vi "Module (Top Level).vi"(8 "error in":errorcluster) -> (0 "error out":errorcluster)   [LabVIEW 2017, in "Controller.lvlib"]
uses:
  Controller.lvlib
  User Events/TypeDefs/Shutdown UE FGV Command.ctl
  Global TypeDefs/Registered Modules.ctl
  Private TypeDefs/Messages.ctl
  Game/Public TypeDefs/Messages.ctl
  mypam/Public TypeDefs/Messages.ctl
  winhost/Public TypeDefs/Messages.ctl
  Private TypeDefs/Event and Data.ctl
  Game/Public TypeDefs/Module Events.ctl
  Game/Libraries/TypeDefs/ClientStatusData.ctl
  mypam/Public TypeDefs/Module Events.ctl
  winhost/Public TypeDefs/Module Events.ctl
  Error Handler/Error Handler.lvlib
  Logger/Logger.lvlib
  Game/Game.lvlib
  mypam/myPAM.lvlib
  WinHost/WinHost.lvlib
  Game/Libraries/GameComms.lvlib
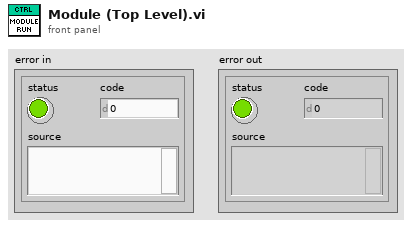
[diagram p1: front panel]
types:
  T1 = typedef "Registered Modules.ctl" = enum16{"Controller", "DAQ", "Error Handler", "Game", "myPAM", "WinHost", "Logger"}
  T2 = typedef "Shutdown UE FGV Command.ctl" = enum16{"create", "get", "destroy"}
  T3 = typedef "WinHost.lvlib/Module Reference.ctl" = cluster{"calling module":T1, "module queues":T4, "module notifiers":T5}
  T4 = typedef "WinHost.lvlib/Module Queues.ctl" = cluster{"message queue":refnum<queue>, "STM queue":refnum<queue>}
  T5 = typedef "WinHost.lvlib/Module Notifiers.ctl" = cluster{"dummy notifier":refnum<notifier>}
  T6 = typedef "myPAM.lvlib/Module Reference.ctl" = cluster{"calling module":T1, "module queues":T7, "module notifiers":T8}
  T7 = typedef "myPAM.lvlib/Module Queues.ctl" = cluster{"message queue":refnum<queue>}
  T8 = typedef "myPAM.lvlib/Module Notifiers.ctl" = cluster{"end eff. pos.":refnum<notifier>}
  T9 = typedef "Game.lvlib/Module Reference.ctl" = cluster{"calling module":T1, "module queues":T10, "module notifiers":T11}
  T10 = typedef "Game.lvlib/Module Queues.ctl" = cluster{"message queue":refnum<queue>}
  T11 = typedef "Game.lvlib/Module Notifiers.ctl" = cluster{"dummy notifier":refnum<notifier>}
  T12 = typedef "Logger.lvlib/Module Reference.ctl" = cluster{"calling module":T1, "module queues":T13, "module notifiers":T14}
  T13 = typedef "Logger.lvlib/Module Queues.ctl" = cluster{"message queue":refnum<queue>}
  T14 = typedef "Logger.lvlib/Module Notifiers.ctl" = cluster{"dummy notifier":refnum<notifier>}
  T15 = typedef "Controller.lvlib/Module Reference.ctl" = cluster{"calling module":T1, "module queues":T16, "module notifiers":T17}
  T16 = typedef "Controller.lvlib/Module Queues.ctl" = cluster{"message queue":refnum<queue>}
  T17 = typedef "Controller.lvlib/Module Notifiers.ctl" = cluster{"dummy notifier":refnum<notifier>}
  T18 = typedef "Error Handler.lvlib/Module Reference.ctl" = cluster{"calling module":T1, "module queues":T19, "module notifiers":T20}
  T19 = typedef "Error Handler.lvlib/Module Queues.ctl" = cluster{"message queue":refnum<queue>}
  T20 = typedef "Error Handler.lvlib/Module Notifiers.ctl" = cluster{"dummy notifier":refnum<notifier>}
  T21 = typedef "Controller.lvlib/Messages.ctl" = enum16{"shutdown", "handle event", "start system"}
  T22 = typedef "myPAM.lvlib/Messages.ctl" = enum16{"calibrate encoders", "enable motors", "disable motors", "operate", "shutdown"}
  T23 = typedef "WinHost.lvlib/Messages.ctl" = enum16{"shutdown", "wait for host", "communicate"}
  T24 = typedef "Game.lvlib/Messages.ctl" = enum16{"wait for client", "communicate", "shutdown"}
  T25 = typedef "Game.lvlib/Module Events.ctl" = enum16{"client connected", "client status change", "client disconnected"}
  T26 = typedef "myPAM.lvlib/Module Events.ctl" = enum16{"critical error"}
  T27 = typedef "WinHost.lvlib/Module Events.ctl" = enum16{"host connected", "enable assistance", "disable assistance", "host disconnected"}
  T28 = typedef "Controller.lvlib/Event and Data.ctl" = cluster{"event":variant, "data":variant}
  T29 = typedef "Game.lvlib/GameComms.lvlib/ClientStatusData.ctl" = cluster{"gameState":u16, "playerName":string, "playerScore":dbl, "gameUnits":string}
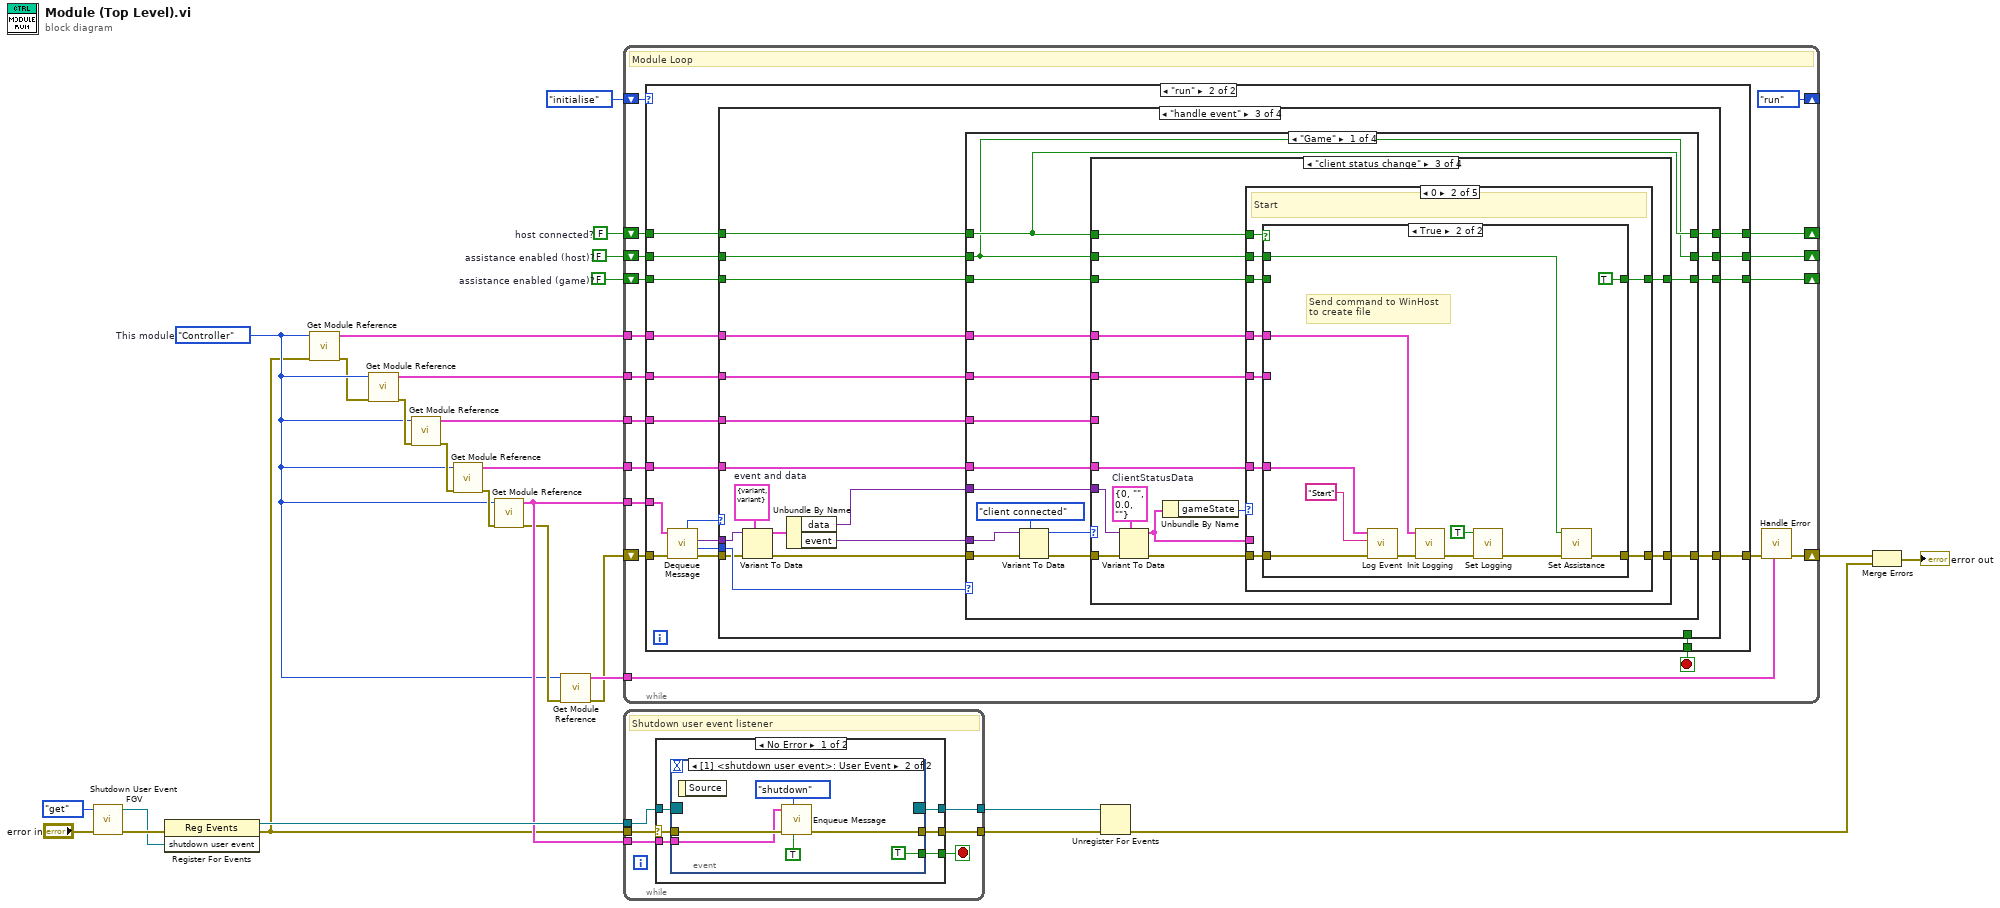
[diagram p0: block diagram]
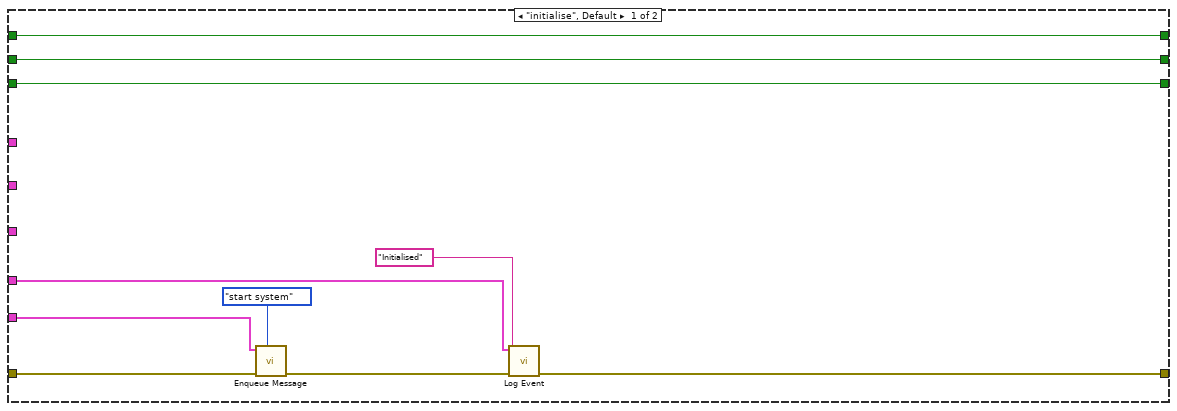
[diagram p2: hidden frame]
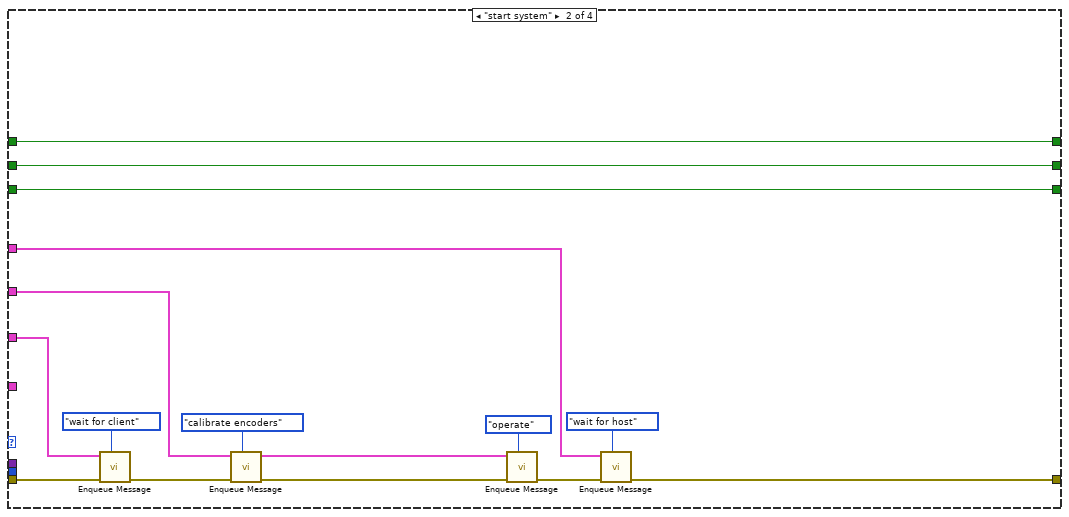
[diagram p4: hidden frame]
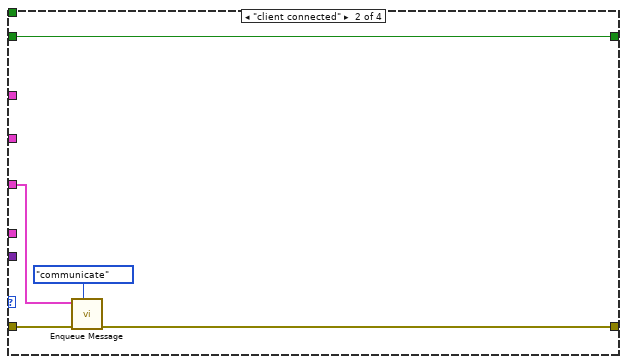
[diagram p6: hidden frame]
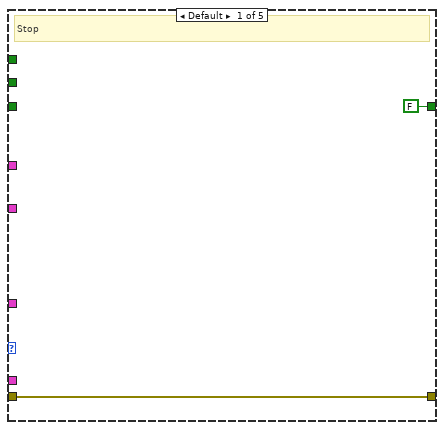
[diagram p7: hidden frame]
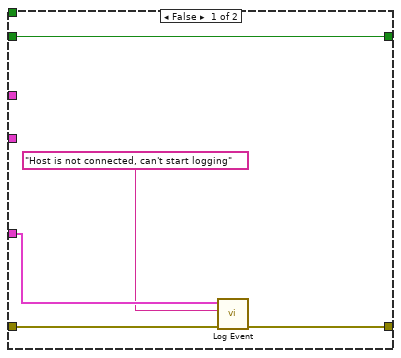
[diagram p8: hidden frame]
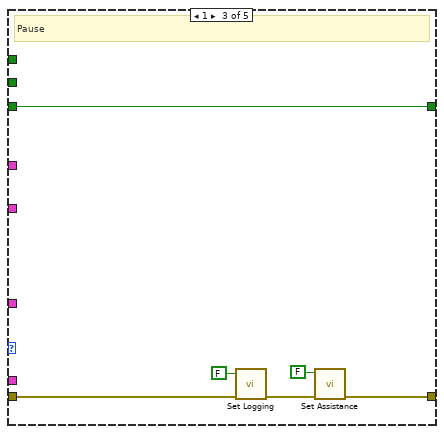
[diagram p9: hidden frame]
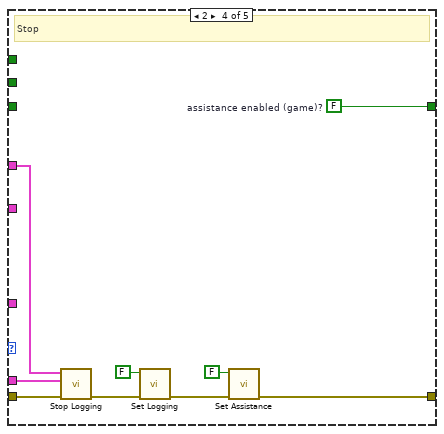
[diagram p10: hidden frame]
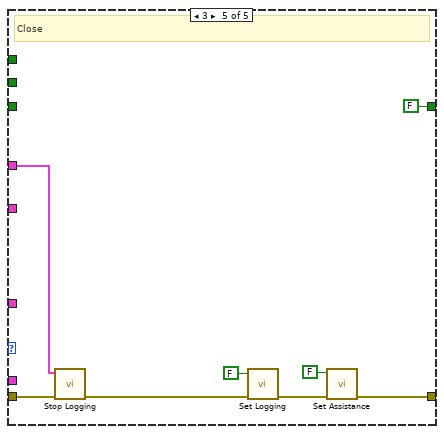
[diagram p11: hidden frame]
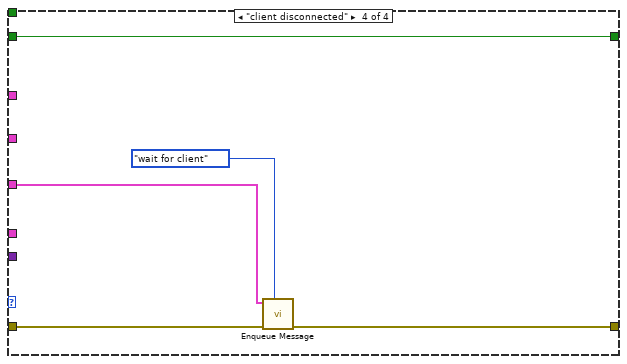
[diagram p12: hidden frame]
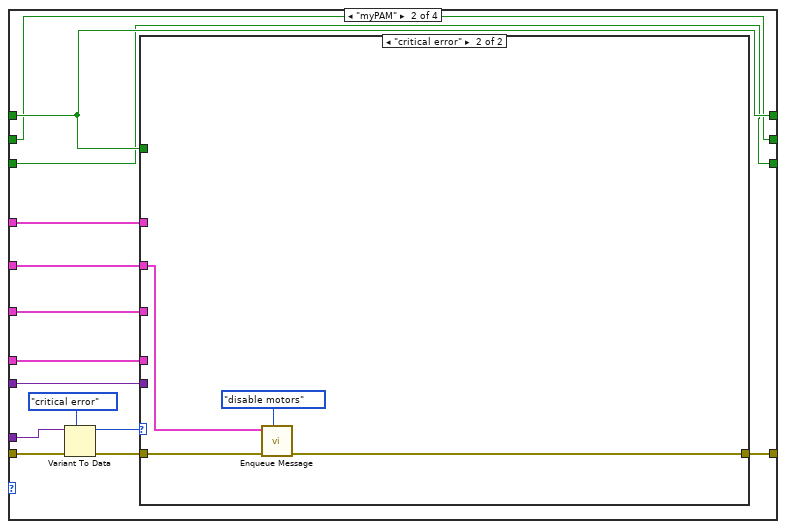
[diagram p13: hidden frame]
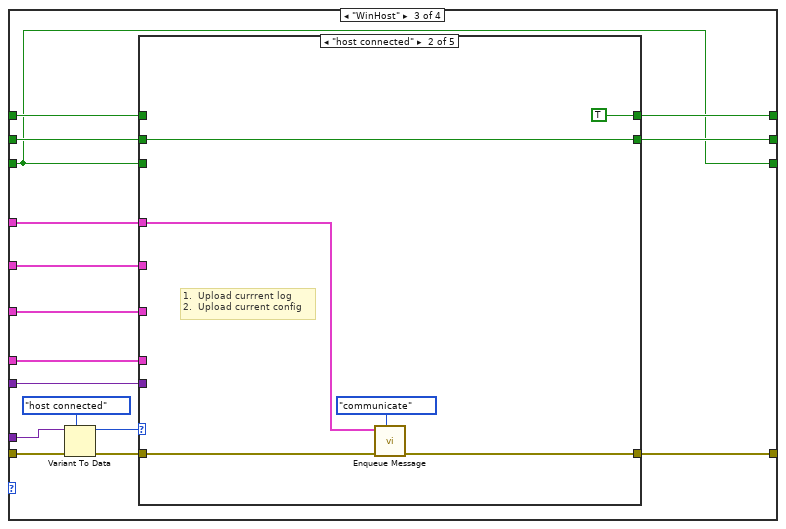
[diagram p15: hidden frame]
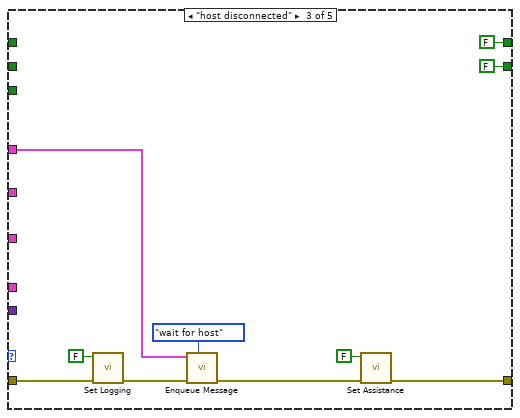
[diagram p17: hidden frame]
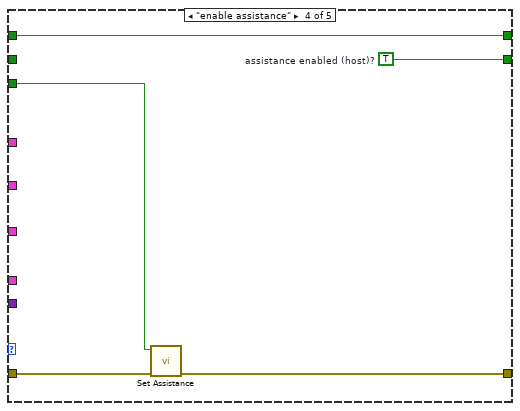
[diagram p18: hidden frame]
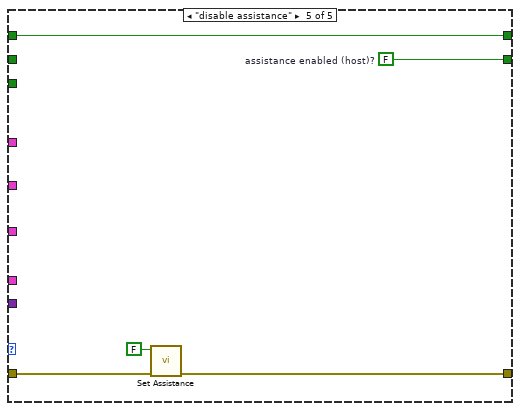
[diagram p19: hidden frame]
diagram:
  w1 = FALSE  # assistance enabled (game)?
  w2 = FALSE  # assistance enabled (host)?
  w4 = FALSE  # host connected?
  w8 = Registered_Modules."Controller"  # This module
  n1 = call "Shutdown User Event FGV.vi"("error in"="error in", "command"=Shutdown_UE_FGV_Command."get" ("Command")) -> ("error out"=w24:errorcluster, "shutdown user event"=w23:refnum<user-event>)  [unwired: 8 in]
  n2 = register-events(error in=w24, w23) -> (reference out=w27:refnum<event-registration>, error out=w7:errorcluster)  [unwired: 1 in]
  n3 = call "Get Module Reference.vi"("error in"=w7, "calling module"=w8) -> ("error out"=w6:errorcluster, "module reference"=w5:T3)  [unwired: 8 in]
  n4 = call "Get Module Reference.vi"("error in"=w6, "calling module"=w8) -> ("error out"=w10:errorcluster, "module reference"=w9:T6)  [unwired: 8 in]
  n5 = call "Get Module Reference.vi"("error in"=w10, "calling module"=w8) -> ("error out"=w12:errorcluster, "module reference"=w11:T9)  [unwired: 8 in]
  n6 = call "Get Module Reference.vi"("error in"=w12, "calling module"=w8) -> ("error out"=w17:errorcluster, "module reference"=w16:T12)  [unwired: 8 in]
  n7 = call "Get Module Reference.vi"("error in"=w17, "calling module"=w8) -> ("error out"=w15:errorcluster, "module reference"=w20:T15)  [unwired: 8 in]
  n8 = call "Get Module Reference.vi"("error in"=w15, "calling module"=w8) -> ("error out"=w13:errorcluster, "module reference"=w14:T18)  [unwired: 8 in]
  n9 = while {
    shift-right: [w40] -> w19
    shift-left: w13 -> [w46]
    tunnel: w20 -> [w45]
    shift-right: [enum16{"initialise", "run"}."run"] -> _
    shift-left: enum16{"initialise", "run"}."initialise" -> [w42]
    tunnel: w16 -> [w39]
    tunnel: w14 -> [w38]
    tunnel: w11 -> [w37]
    tunnel: w9 -> [w36]
    tunnel: w5 -> [w35]
    shift-right: [w33] -> _
    shift-left: w4 -> [w34]
    shift-right: [w32] -> _
    shift-left: w2 -> [w31]
    shift-right: [w29] -> _
    shift-left: w1 -> [w30]
    stop <- w44 stop-if-true
    # "Module Loop"
    n10 = case shown="\"run\"" w42 {
      tunnel: [w51 w74] -> w41
      tunnel: w45 -> [w54 w72]
      tunnel: [_ w68] -> w44
      tunnel: w46 -> [w53 w73]
      tunnel: w39 -> [w55 w67]
      tunnel: w37 -> [_ w65]
      tunnel: w36 -> [_ w64]
      tunnel: w35 -> [_ w63]
      tunnel: w34 -> [w49 w62]
      tunnel: [w49 w61] -> w33
      tunnel: [w48 w60] -> w32
      tunnel: w31 -> [w48 w59]
      tunnel: w30 -> [w47 w58]
      tunnel: [w47 w57] -> w29
      frame "initialise", Default {
        n11 = call "Enqueue Message.vi"("message"=Messages."start system", "error in"=w53, "module reference in"=w54) -> ("error out"=w52:errorcluster)  [unwired: 7 in, 1 out]
        n12 = call "Log Event.vi"("error in"=w52, "event"="Initialised" ("string"), "module reference in"=w55) -> ("error out"=w51:errorcluster)  [unwired: 7 in, 1 out]
      }
      frame "run" {
        n13 = call "Dequeue Message.vi"("error in"=w73, "module reference in"=w72) -> ("error out"=w70:errorcluster, "source"=w69:T1, "data"=w66:variant, "message"=w71:T21)  [unwired: 5 in, 1 out]
        n14 = case shown="\"handle event\"" w71 {
          tunnel: [w78 w86 w112 w277] -> w74
          tunnel: w70 -> [w78 w94 w109 w277]
          tunnel: w66 -> [_ _ w110 _]
          tunnel: w69 -> [_ _ w113 _]
          tunnel: [_ _ _ TRUE] -> w68
          tunnel: w67 -> [_ _ w103 _]
          tunnel: w65 -> [_ w93 w105 _]
          tunnel: w64 -> [_ w89 w101 _]
          tunnel: w63 -> [_ w87 w100 _]
          tunnel: w62 -> [w77 w85 w102 w275]
          tunnel: [w77 w85 w99 w275] -> w61
          tunnel: [w76 w82 w98 w274] -> w60
          tunnel: w59 -> [w76 w82 w97 w274]
          tunnel: w58 -> [w75 w81 w96 w273]
          tunnel: [w75 w81 w95 w273] -> w57
          frame Default {
          }
          frame "start system" {
            n15 = call "Enqueue Message.vi"("message"=Messages."wait for client", "error in"=w94, "module reference in"=w93) -> ("error out"=w91:errorcluster)  [unwired: 7 in, 1 out]
            n16 = call "Enqueue Message.vi"("message"=Messages."calibrate encoders", "error in"=w91, "module reference in"=w89) -> ("error out"=w80:errorcluster, "module reference out"=w79:T6)  [unwired: 7 in]
            n17 = call "Enqueue Message.vi"("message"=Messages."operate", "error in"=w80, "module reference in"=w79) -> ("error out"=w83:errorcluster)  [unwired: 7 in, 1 out]
            n18 = call "Enqueue Message.vi"("message"=Messages."wait for host", "error in"=w83, "module reference in"=w87) -> ("error out"=w86:errorcluster)  [unwired: 7 in, 1 out]
          }
          frame "handle event" {
            w111 = T28 {"event"=variant, "data"=variant}  # event and data
            n19 = Variant To Data(error in=w109, type=w111, Variant=w110) -> (data=w107:T28, error out=w108:errorcluster)
            n20 = Unbundle By Name(w107) -> ("data"=w104:variant, "event"=w106:variant)
            n21 = case shown="\"Game\"" w113 {
              tunnel: w108 -> [w126 w217 w238 w272]
              tunnel: [w123 w214 w227 w272] -> w112
              tunnel: w106 -> [w127 w218 w239 _]
              tunnel: w105 -> [w125 w216 w237 _]
              tunnel: w104 -> [w122 w213 w235 _]
              tunnel: w103 -> [w120 w211 w233 _]
              tunnel: w102 -> [w119 w210 w232 w271]
              tunnel: w101 -> [w118 w209 w231 _]
              tunnel: w100 -> [w117 w208 w230 _]
              tunnel: [w119 w210 w228 w271] -> w99
              tunnel: [w116 w206 w226 w270] -> w98
              tunnel: w97 -> [w116 w206 w225 w270]
              tunnel: w96 -> [w115 w205 w224 w269]
              tunnel: [w114 w205 w224 w269] -> w95
              frame "Game" {
                n22 = Variant To Data(error in=w126, type=Module_Events."client connected" ("module events"), Variant=w127) -> (data=w124:T25, error out=w121:errorcluster)
                n23 = case shown="\"client status change\"" w124 {
                  tunnel: w125 -> [_ w133 _ w201]
                  tunnel: w121 -> [w130 w135 w149 w203]
                  tunnel: [w130 w134 w144 w202] -> w123
                  tunnel: w122 -> [_ _ w148 _]
                  tunnel: w120 -> [_ _ w140 _]
                  tunnel: w119 -> [_ _ w143 _]
                  tunnel: w118 -> [_ _ w141 _]
                  tunnel: w117 -> [_ _ w142 _]
                  tunnel: w116 -> [_ _ w138 _]
                  tunnel: w115 -> [w129 w131 w137 w200]
                  tunnel: [w129 w131 w136 w200] -> w114
                  frame Default {
                  }
                  frame "client connected" {
                    n24 = call "Enqueue Message.vi"("message"=Messages."communicate", "error in"=w135, "module reference in"=w133) -> ("error out"=w134:errorcluster)  [unwired: 7 in, 1 out]
                  }
                  frame "client status change" {
                    w147 = T29 {"gameState"=0, "playerName"="", "playerScore"=0.0, "gameUnits"=""}  # ClientStatusData
                    n25 = Variant To Data(error in=w149, type=w147, Variant=w148) -> (data=w139:T29, error out=w146:errorcluster)
                    n26 = Unbundle By Name(w139) -> ("gameState"=w145:u16)
                    n27 = case shown="0" w145 {
                      tunnel: w146 -> [w151 w159 w182 w191 w197]
                      tunnel: [w151 w158 w178 w184 w193] -> w144
                      tunnel: w143 -> [_ w160 _ _ _]
                      tunnel: w142 -> [_ w157 _ w190 w196]
                      tunnel: w141 -> [_ w156 _ _ _]
                      tunnel: w140 -> [_ w155 _ _ _]
                      tunnel: w139 -> [_ _ _ w189 _]
                      tunnel: w138 -> [_ w154 _ _ _]
                      tunnel: w137 -> [_ w153 w177 _ _]
                      tunnel: [FALSE ("assistance enabled (game)?") w152 w177 w183 FALSE ("assistance enabled (game)?")] -> w136
                      frame Default {
                        # "Stop"
                      }
                      frame 0 {
                        # "Start"
                        n28 = case shown="True" w160 {
                          tunnel: w159 -> [w165 w174]
                          tunnel: [w162 w168] -> w158
                          tunnel: w157 -> [_ w175]
                          tunnel: w156 -> [_ _]
                          tunnel: w155 -> [w164 w172]
                          tunnel: w154 -> [_ w167]
                          tunnel: w153 -> [w161 _]
                          tunnel: [w161 TRUE ("assistance enabled (game)?")] -> w152
                          frame False {
                            n29 = call "Log Event.vi"("error in"=w165, "event"="Host is not connected, can't start logging", "module reference in"=w164) -> ("error out"=w162:errorcluster)  [unwired: 7 in, 1 out]
                          }
                          frame True {
                            # "Send command to WinHost\nto create file"
                            n30 = call "Log Event.vi"("error in"=w174, "event"="Start", "module reference in"=w172) -> ("error out"=w173:errorcluster)  [unwired: 7 in, 1 out]
                            n31 = call "Init Logging.vi"("error in"=w173, "module reference in"=w175) -> ("error out"=w176:errorcluster)  [unwired: 8 in, 1 out]
                            n32 = call "Set Logging.vi"("error in"=w176, "log?"=TRUE) -> ("error out"=w169:errorcluster)  [unwired: 9 in]
                            n33 = call "Set Assistance.vi"("error in"=w169, "assistance?"=w167) -> ("error out"=w168:errorcluster)  [unwired: 9 in]
                          }
                        }
                      }
                      frame 1 {
                        # "Pause"
                        n34 = call "Set Logging.vi"("error in"=w182, "log?"=FALSE) -> ("error out"=w179:errorcluster)  [unwired: 9 in]
                        n35 = call "Set Assistance.vi"("error in"=w179, "assistance?"=FALSE) -> ("error out"=w178:errorcluster)  [unwired: 9 in]
                      }
                      frame 2 {
                        w183 = FALSE  # assistance enabled (game)?
                        # "Stop"
                        n36 = call "Stop Logging.vi"("error in"=w191, "gameStatus"=w189, "module reference in"=w190) -> ("error out"=w188:errorcluster)  [unwired: 7 in, 1 out]
                        n37 = call "Set Logging.vi"("error in"=w188, "log?"=FALSE) -> ("error out"=w185:errorcluster)  [unwired: 9 in]
                        n38 = call "Set Assistance.vi"("error in"=w185, "assistance?"=FALSE) -> ("error out"=w184:errorcluster)  [unwired: 9 in]
                      }
                      frame 3 {
                        # "Close"
                        n39 = call "Stop Logging.vi"("error in"=w197, "module reference in"=w196) -> ("error out"=w195:errorcluster)  [unwired: 8 in, 1 out]
                        n40 = call "Set Logging.vi"("error in"=w195, "log?"=FALSE) -> ("error out"=w194:errorcluster)  [unwired: 9 in]
                        n41 = call "Set Assistance.vi"("error in"=w194, "assistance?"=FALSE) -> ("error out"=w193:errorcluster)  [unwired: 9 in]
                      }
                    }
                  }
                  frame "client disconnected" {
                    n42 = call "Enqueue Message.vi"("message"=Messages."wait for client", "error in"=w203, "module reference in"=w201) -> ("error out"=w202:errorcluster)  [unwired: 7 in, 1 out]
                  }
                }
              }
              frame "myPAM" {
                n43 = Variant To Data(error in=w217, type=Module_Events."critical error" ("module events"), Variant=w218) -> (data=w215:T26, error out=w212:errorcluster)
                n44 = case shown="\"critical error\"" w215 {
                  tunnel: w216 -> [_ _]
                  tunnel: w212 -> [w219 w223]
                  tunnel: [w219 w220] -> w214
                  tunnel: w213 -> [_ _]
                  tunnel: w211 -> [_ _]
                  tunnel: w210 -> [_ _]
                  tunnel: w209 -> [_ w222]
                  tunnel: w208 -> [_ _]
                  frame Default {
                  }
                  frame "critical error" {
                    n45 = call "Enqueue Message.vi"("message"=Messages."disable motors", "error in"=w223, "module reference in"=w222) -> ("error out"=w220:errorcluster)  [unwired: 7 in, 1 out]
                  }
                }
              }
              frame "WinHost" {
                n46 = Variant To Data(error in=w238, type=Module_Events."host connected" ("module events"), Variant=w239) -> (data=w236:T27, error out=w234:errorcluster)
                n47 = case shown="\"host connected\"" w236 {
                  tunnel: w237 -> [_ _ _ _ _]
                  tunnel: w234 -> [w242 w247 w254 w262 w267]
                  tunnel: [w242 w246 w249 w260 w264] -> w227
                  tunnel: w235 -> [_ _ _ _ _]
                  tunnel: w233 -> [_ _ _ _ _]
                  tunnel: w232 -> [w241 _ _ w263 w268]
                  tunnel: w231 -> [_ _ _ _ _]
                  tunnel: w230 -> [_ w245 w256 _ _]
                  tunnel: [w241 TRUE FALSE ("Host connected?") w263 w268] -> w228
                  tunnel: [w240 w243 FALSE ("assistance enabled (host)?") w261 w265] -> w226
                  tunnel: w225 -> [w240 w243 _ _ _]
                  tunnel: w224 -> [_ _ _ w259 _]
                  frame Default {
                  }
                  frame "host connected" {
                    # "1.  Upload currrent log\n2.  Upload current config"
                    n48 = call "Enqueue Message.vi"("message"=Messages."communicate", "error in"=w247, "module reference in"=w245) -> ("error out"=w246:errorcluster)  [unwired: 7 in, 1 out]
                  }
                  frame "host disconnected" {
                    n49 = call "Set Logging.vi"("error in"=w254, "log?"=FALSE) -> ("error out"=w253:errorcluster)  [unwired: 9 in]
                    n50 = call "Enqueue Message.vi"("message"=Messages."wait for host", "error in"=w253, "module reference in"=w256) -> ("error out"=w251:errorcluster)  [unwired: 7 in, 1 out]
                    n51 = call "Set Assistance.vi"("error in"=w251, "assistance?"=FALSE) -> ("error out"=w249:errorcluster)  [unwired: 9 in]
                  }
                  frame "enable assistance" {
                    w261 = TRUE  # assistance enabled (host)?
                    n52 = call "Set Assistance.vi"("error in"=w262, "assistance?"=w259) -> ("error out"=w260:errorcluster)  [unwired: 9 in]
                  }
                  frame "disable assistance" {
                    w265 = FALSE  # assistance enabled (host)?
                    n53 = call "Set Assistance.vi"("error in"=w267, "assistance?"=FALSE) -> ("error out"=w264:errorcluster)  [unwired: 9 in]
                  }
                }
              }
              frame Default {
              }
            }
          }
          frame "shutdown" {
          }
        }
      }
    }
    n54 = call "Handle Error.vi"("module reference in"=w38, "error in"=w41) -> ("error out"=w40:errorcluster)  [unwired: 9 in]
  }
  n55 = while {
    tunnel: w27 -> [w283]
    tunnel: [w282] -> w26
    tunnel: w7 -> [w280]
    tunnel: [w279] -> w22
    tunnel: w20 -> [w278]
    stop <- w281 stop-if-true
    # "Shutdown user event listener"
    n56 = case shown="No Error" w280 {
      selector: w280 -> [w286 _]
      tunnel: w283 -> [w289 w298]
      tunnel: [w288 w298] -> w282
      tunnel: [w287 TRUE] -> w281
      tunnel: [w285 errorcluster {"status"=FALSE, "code"=0, "source"=""} ("error out")] -> w279
      tunnel: w278 -> [w284 _]
      frame No Error {
        n57 = event shown="[1] <shutdown user event>: User Event" {
          selector: w289 -> [_ _]
          dyn-events: [_ _] -> w288
          timeout: _ -> [_ _]
          tunnel: w286 -> [w290 w294]
          tunnel: [w290 w293] -> w285
          tunnel: [_ TRUE] -> w287
          tunnel: w284 -> [_ w292]
          event Timeout {
            n58 = event-data() -> ()  [unwired: 1 in, 3 out]
          }
          event User Event {
            n59 = event-data() -> ()  [unwired: 1 in, 1 out]
            n60 = call "Enqueue Message.vi"("high priority"=TRUE, "message"=Messages."shutdown", "error in"=w294, "module reference in"=w292) -> ("error out"=w293:errorcluster)  [unwired: 6 in, 1 out]
          }
        }
      }
      frame Error {
      }
    }
  }
  n61 = Unregister For Events(event registration refnum=w26, error in=w22) -> (error out=w3:errorcluster)
  n62 = Merge Errors(w19, w3) -> (→"error out":errorcluster)
